vi "pratik2-case1.vi"(11 "Cluster 11":T1) -> (1 "number 5":u32 format="%02x", 2 "number 4":u32 format="%x", 3 "appended array 4":bool[](array[boolean]), 4 "appended array 5":bool[](array[boolean]), 5 "appended array 6":bool[](array[boolean]), 6 "number 6":u32 format="%02x")   [LabVIEW 2024]
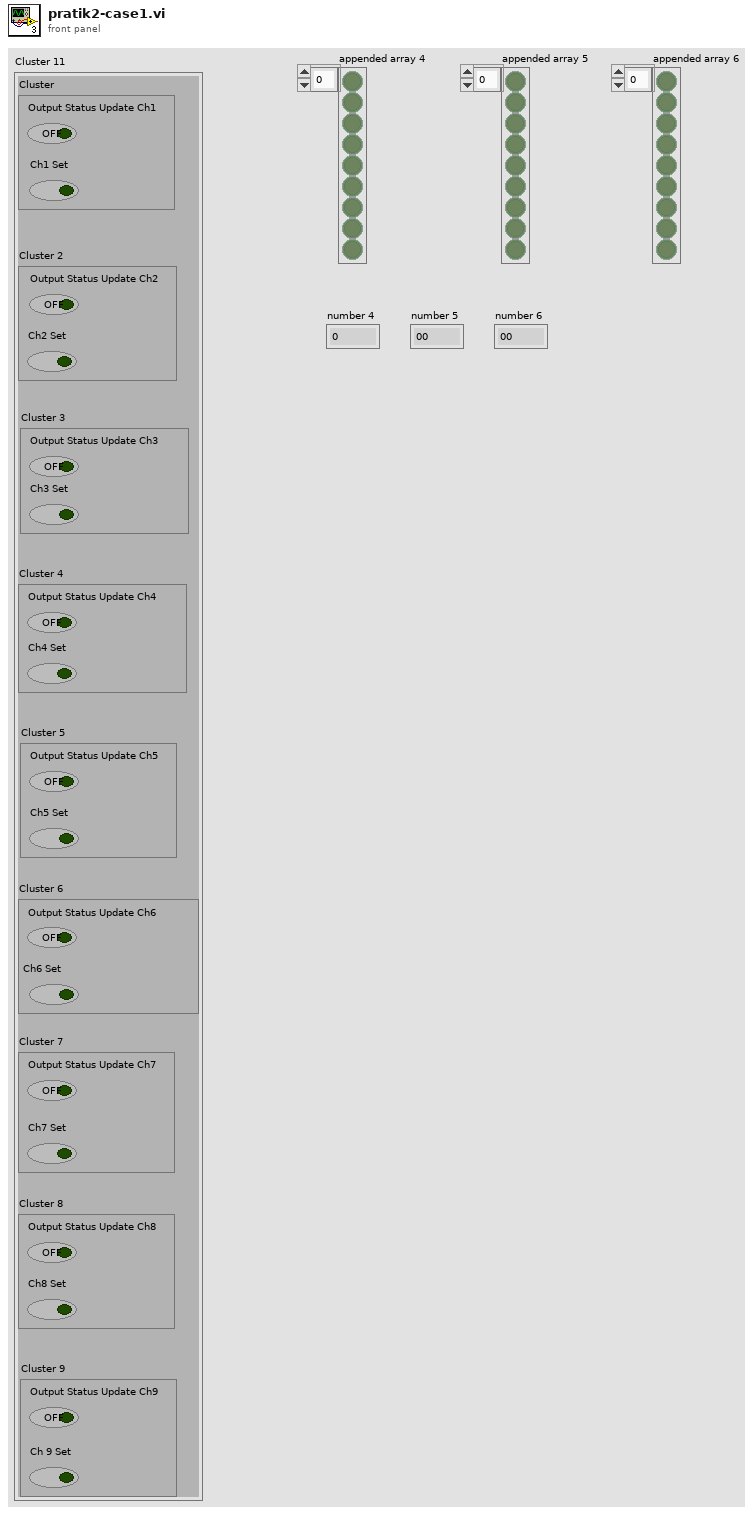
[diagram p1: front panel]
types:
  T1 = cluster{"Cluster":cluster{"Output Status Update Ch1":bool, "Ch1 Set":bool}, "Cluster 2":cluster{"Output Status Update Ch2":bool, "Ch2 Set":bool}, "Cluster 3":cluster{"Ch3 Set":bool, "Output Status Update Ch3":bool}, "Cluster 4":cluster{"Ch4 Set":bool, "Output Status Update Ch4":bool}, "Cluster 5":cluster{"Ch5 Set":bool, "Output Status Update Ch5":bool}, "Cluster 6":cluster{"Ch6 Set":bool, "Output Status Update Ch6":bool}, "Cluster 7":cluster{"Ch7 Set":bool, "Output Status Update Ch7":bool}, "Cluster 8":cluster{"Ch8 Set":bool, "Output Status Update Ch8":bool}, "Cluster 9":cluster{"Ch 9 Set":bool, "Output Status Update Ch9":bool}}
  T2 = cluster{"Output Status Update Ch1":bool, "Ch1 Set":bool}
  T3 = cluster{"Output Status Update Ch2":bool, "Ch2 Set":bool}
  T4 = cluster{"Ch3 Set":bool, "Output Status Update Ch3":bool}
  T5 = cluster{"Ch4 Set":bool, "Output Status Update Ch4":bool}
  T6 = cluster{"Ch5 Set":bool, "Output Status Update Ch5":bool}
  T7 = cluster{"Ch6 Set":bool, "Output Status Update Ch6":bool}
  T8 = cluster{"Ch7 Set":bool, "Output Status Update Ch7":bool}
  T9 = cluster{"Ch8 Set":bool, "Output Status Update Ch8":bool}
  T10 = cluster{"Ch 9 Set":bool, "Output Status Update Ch9":bool}
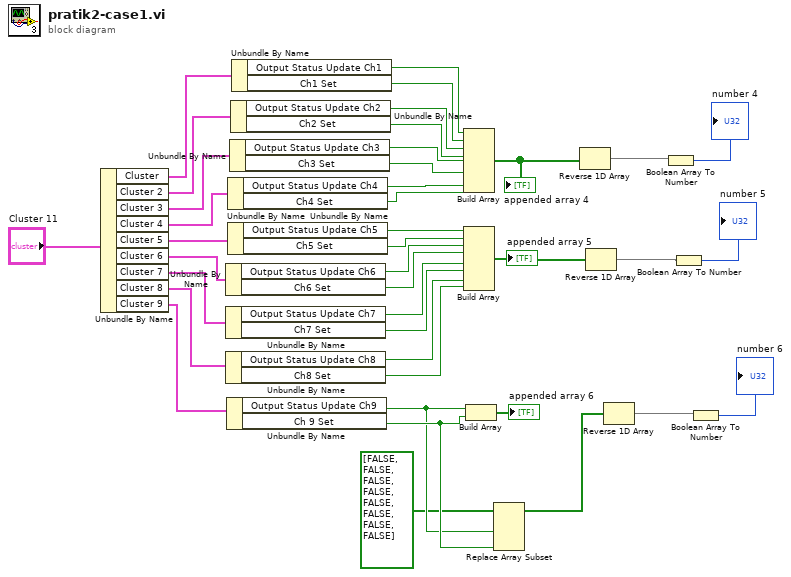
[diagram p0: block diagram]
diagram:
  n1 = Unbundle By Name("Cluster 11") -> ("Cluster"=w2:T2, "Cluster 2"=w3:T3, "Cluster 3"=w4:T4, "Cluster 4"=w5:T5, "Cluster 5"=w6:T6, "Cluster 6"=w7:T7, "Cluster 7"=w8:T8, "Cluster 8"=w9:T9, "Cluster 9"=w10:T10)
  n2 = Unbundle By Name(w7) -> ("Output Status Update Ch6"=w21:bool, "Ch6 Set"=w22:bool)
  n3 = Unbundle By Name(w8) -> ("Output Status Update Ch7"=w23:bool, "Ch7 Set"=w24:bool)
  n4 = Unbundle By Name(w9) -> ("Output Status Update Ch8"=w25:bool, "Ch8 Set"=w26:bool)
  n5 = Unbundle By Name(w10) -> ("Output Status Update Ch9"=w33:bool, "Ch 9 Set"=w34:bool)
  n6 = Unbundle By Name(w5) -> ("Output Status Update Ch4"=w17:bool, "Ch4 Set"=w18:bool)
  n7 = Unbundle By Name(w6) -> ("Output Status Update Ch5"=w19:bool, "Ch5 Set"=w20:bool)
  n8 = Unbundle By Name(w4) -> ("Output Status Update Ch3"=w15:bool, "Ch3 Set"=w16:bool)
  n9 = Unbundle By Name(w3) -> ("Output Status Update Ch2"=w13:bool, "Ch2 Set"=w14:bool)
  n10 = Unbundle By Name(w2) -> ("Output Status Update Ch1"=w11:bool, "Ch1 Set"=w12:bool)
  n11 = Build Array "Build Array"(w11, w12, w13, w14, w15, w16, w17, w18) -> (w27:bool[])
  "appended array 4" <- w27
  n12 = Build Array "Build Array"(w19, w20, w21, w22, w23, w24, w25, w26) -> (w29:bool[])
  "appended array 5" <- w29
  n13 = Build Array "Build Array"(w33, w34) -> (→"appended array 6":bool[])
  n14 = Replace Array Subset "Replace Array Subset"(array=bool[] [FALSE, FALSE, FALSE, FALSE, FALSE, FALSE, FALSE, FALSE] ("appended array 6"), new element #1=w33, new element #2=w34) -> (w36:bool[])  [unwired: 2 in]
  n15 = Reverse 1D Array(array=w27) -> (reversed array=w28:bool[])
  n16 = Reverse 1D Array(array=w29) -> (reversed array=w30:bool[])
  n17 = Reverse 1D Array(array=w36) -> (reversed array=w31:bool[])
  n18 = Boolean Array To Number(Boolean array=w28) -> (number=→"number 4":u32)
  n19 = Boolean Array To Number(Boolean array=w30) -> (number=→"number 5":u32)
  n20 = Boolean Array To Number(Boolean array=w31) -> (number=→"number 6":u32)
